vi "Choosed_Input_to_Array.vi"(8 "error in (no error)":errorcluster, 11 "UI_Cluster_In":T1) -> (0 "error out":errorcluster, 3 "UI_Cluster_Out":T1)   [LabVIEW 2020]
uses:
  controls/UI_Ref_Cluster.ctl
  07e20563-7f03-42b7-a7af-6da6fdcb7415.vi
  a8c2a786-0aa3-48dd-9beb-02b2d9557022.vi
  a1dbc9c5-7b35-4c23-a05a-33ad56e800fb.vi
  <vilib>/Comparison/Less/Less Functor/Less Functor.lvclass
  <vilib>/Comparison/Equal/Equal Functor/Equal Functor.lvclass
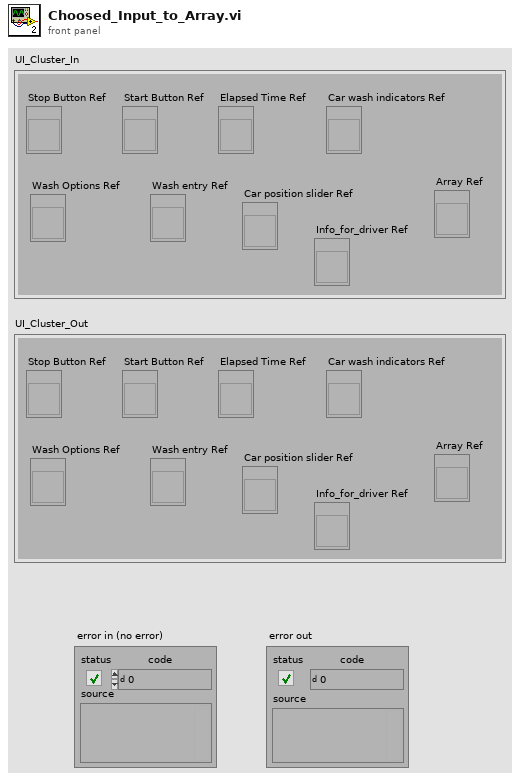
[diagram p1: front panel]
types:
  T1 = typedef "UI_Ref_Cluster.ctl" = cluster{"Stop Button Ref":refnum<vi>, "Start Button Ref":refnum<vi>, "Elapsed Time Ref":refnum<vi>, "Car wash indicators Ref":refnum<vi>, "Wash Options Ref":refnum<vi>, "Wash entry Ref":refnum<vi>, "Car position slider Ref":refnum<vi>, "Info_for_driver Ref":refnum<vi>, "Array Ref":refnum<vi>}
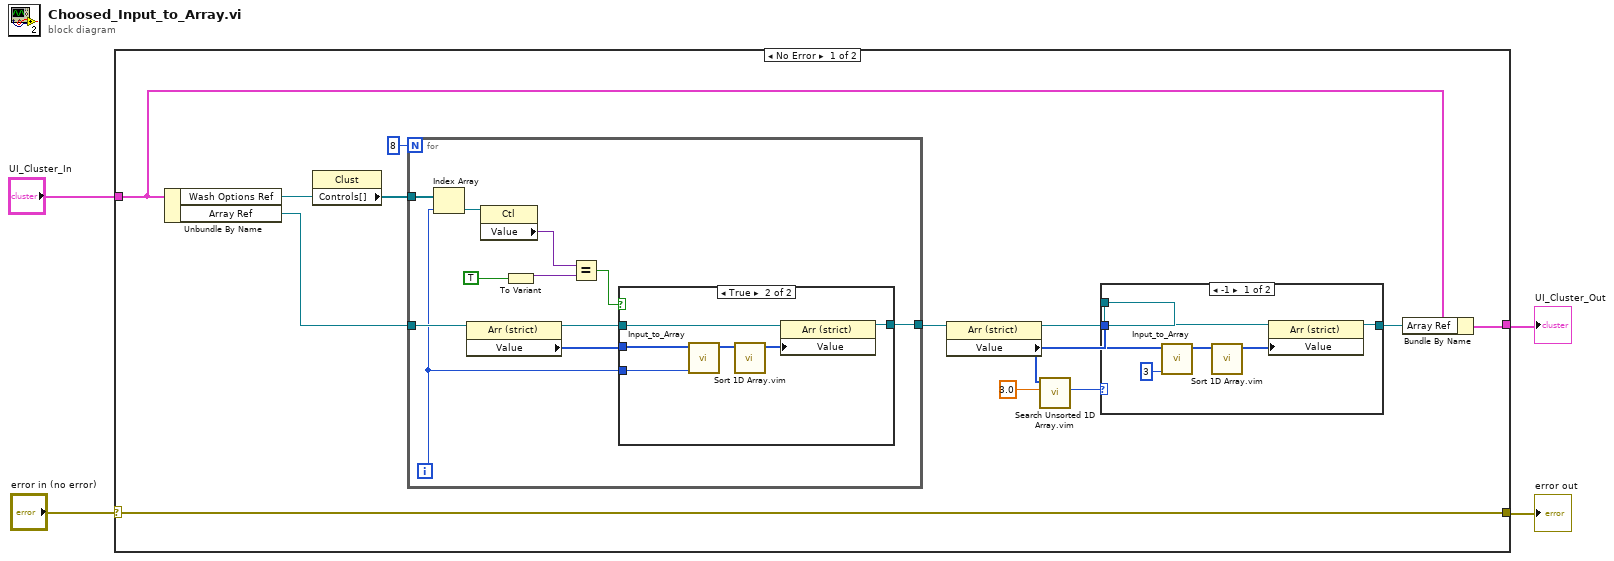
[diagram p0: block diagram]
diagram:
  n1 = case shown="No Error" "error in (no error)" {
    selector: "error in (no error)" -> [w12 w44]
    tunnel: [w12 w44] -> w3
    tunnel: "UI_Cluster_In" -> [w13 w43]
    tunnel: [w6 w43] -> w1
    frame No Error {
      n2 = Unbundle By Name(w13) -> ("Wash Options Ref"=w17:refnum<vi>, "Array Ref"=w14:refnum<vi>)
      n3 = property class="Clust"(reference=w17) -> ("Controls[]"=w15:refnum<vi>[])  [unwired: 1 in, 2 out]
      n4 = for {
        N: 8 -> [_]
        tunnel: w15 -> [w35]
        tunnel: w14 -> [w30]
        tunnel: [w26] -> w11
        i -> [w28]
        n5 = Index Array(array=w35, index=w28) -> (element=w34:refnum<vi>)
        n6 = property class="Arr (strict)"(reference=w30) -> (reference out=w27:refnum<vi>, "Value"=w29:i8[])  [unwired: 1 in, 1 out]
        n7 = property class="Ctl"(reference=w34) -> ("Value"=w33:variant)  [unwired: 1 in, 2 out]
        n8 = To Variant(anything=TRUE) -> (Variant=w25:variant)
        n9 = Equal?(x=w33, y=w25) -> (x = y?=w31:bool)
        n10 = case shown="True" w31 {
          tunnel: w29 -> [_ w41]
          tunnel: w28 -> [_ w40]
          tunnel: w27 -> [w36 w39]
          tunnel: [w36 w38] -> w26
          frame False {
          }
          frame True {
            n11 = call "Input_to_Array.vi"("Numeric"=w40, "Array_In"=w41) -> ("Array_Out"=w42:i8[])  [unwired: 9 in]
            n12 = call "Sort 1D Array.vim"("unsorted array"=w42) -> ("sorted array"=w37:i8[])  [unwired: 10 in]
            n13 = property class="Arr (strict)"(reference=w39, "Value"=w37) -> (reference out=w38:refnum<vi>)  [unwired: 1 in, 1 out]
          }
        }
      }
      n14 = property class="Arr (strict)"(reference=w11) -> (reference out=w9:refnum<vi>, "Value"=w8:i8[])  [unwired: 1 in, 1 out]
      n15 = call "Search Unsorted 1D Array.vim"("element"=3.0, "unsorted 1D array"=w8) -> ("index of element"=w5:i32)  [unwired: 9 in]
      n16 = case shown="-1" w5 {
        tunnel: w8 -> [w23 _]
        tunnel: w9 -> [w20 w24]
        tunnel: [w18 w24] -> w7
        frame -1 {
          n17 = call "Input_to_Array.vi"("Numeric"=i8 3, "Array_In"=w23) -> ("Array_Out"=w21:i8[])  [unwired: 9 in]
          n18 = call "Sort 1D Array.vim"("unsorted array"=w21) -> ("sorted array"=w19:i8[])  [unwired: 10 in]
          n19 = property class="Arr (strict)"(reference=w20, "Value"=w19) -> (reference out=w18:refnum<vi>)  [unwired: 1 in, 1 out]
        }
        frame Default {
        }
      }
      n20 = Bundle By Name(cluster=w13, "Array Ref"=w7) -> (w6:T1)
    }
    frame Error {
    }
  }
  "UI_Cluster_Out" <- w1
  "error out" <- w3
